vi "lvstyx_read_all_path.vi"(7 "Log? (T)":bool=TRUE, 8 "error in (no error)":errorcluster, 9 "path":string, 10 "lim":i32=2048, 11 "client ptr":u32) -> (0 "error out":errorcluster, 2 "buf":string, 3 "dup client ptr":u32)   [LabVIEW 2010, in "lib1299.lvlib"]
uses:
  lib1299.lvlib
  cstyx/win32/cstyx.dll
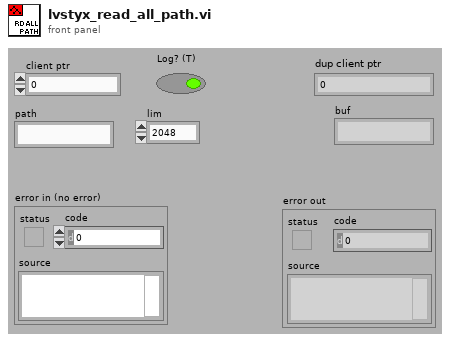
[diagram p1: front panel]
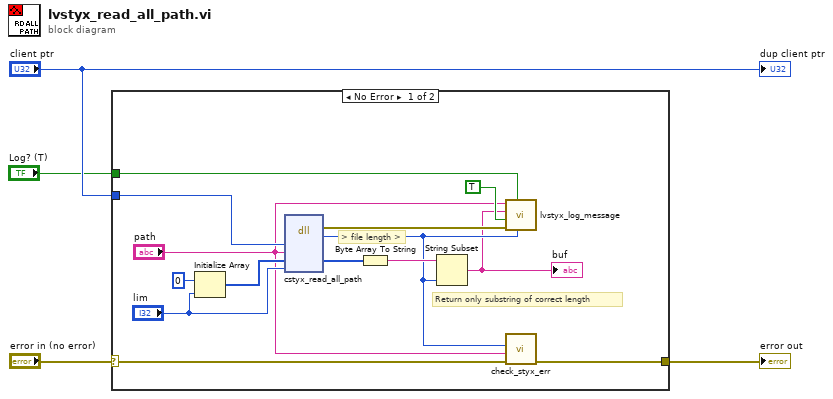
[diagram p0: block diagram]
diagram:
  n1 = case shown="No Error" "error in (no error)" {
    selector: "error in (no error)" -> [w12 w19]
    tunnel: "client ptr" -> [w16 _]
    tunnel: [w15 w19] -> w4
    tunnel: "Log? (T)" -> [w9 _]
    frame No Error {
      # "Return only substring of correct length"
      # "> file length >"
      n2 = Initialize Array(i8 0 ("element"), "lim") -> (w14:i8[])
      n3 = dll-call lib="C:/work/ads1299evm/lib_1299/Styx/cstyx/win32/cstyx.dll" fn="cstyx_read_all_path"("client"=w16, "path"="path", "buf"=w14, "lim"="lim") -> (error out=w11:errorcluster, w7:i32, "buf"=w13:i8[])  [unwired: 6 in, 1 out]
      n4 = Byte Array To String(unsigned byte array=w13) -> (string=w8:string)
      n5 = String Subset(string=w8, length (rest)=w7) -> (substring=w6:string)  [unwired: 1 in]
      "buf" <- w6
      n6 = call "lvstyx_log_message.vi"("File Length"=w7, "Logging Enable (T)"=w9, "error in (no error)"=w11, "Read? (F)"=TRUE, "File value"=w6, "File Name"="path") -> ()  [unwired: 5 in, 1 out]
      n7 = call "check_styx_err.vi"("error in (no error)"=w12, "Additional Comment"="path", "return val"=w7) -> ("error out"=w15:errorcluster)  [unwired: 8 in]
    }
    frame Error {
    }
  }
  "error out" <- w4
  "dup client ptr" <- "client ptr"
